vi "swissCryoMonCtrl.vi"() -> ()   [LabVIEW 2012]
uses:
  <instrlib>/Lake Shore Cryotronics 340/Lake Shore Cryotronics 340.lvlib
panel:
  in  "VISA resource name":refnum<visa-resource-name>
  # "SwissCryoStat Monitor"
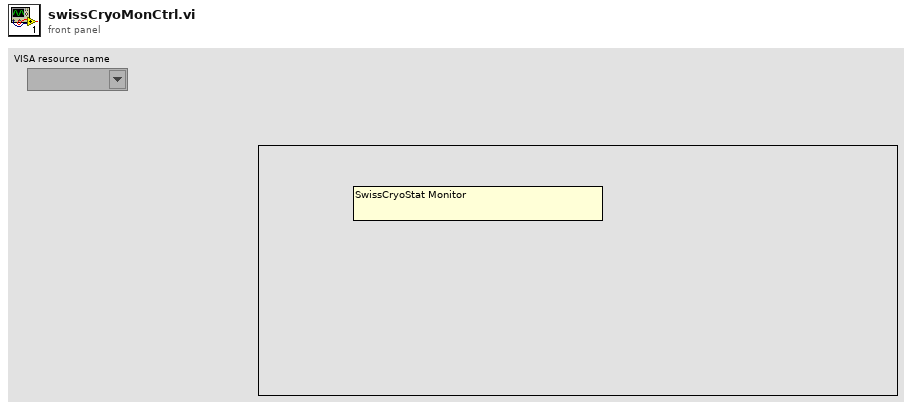
[diagram p1: front panel]
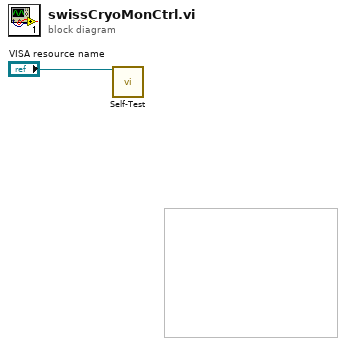
[diagram p0: block diagram]
diagram:
  n1 = call <instrlib>:"Self-Test.vi"("VISA resource name"="VISA resource name") -> ()  [unwired: 11 in, 4 out]
